vi "peak -- four corner circle transformation logic.vi"(6 "corrected phase":dbl, 7 "4 corner circle transformation":T3=enum."fix phase", 8 "lorentzian in":T1 {"z∞ (V)" format="%#9_9f"; "Q" format="%#9_9f"; "φ (rad)" format="%#9_9f"; "Γ (Hz)" format="%#9_9f"; "f (Hz)" format="%#9_9f"}, 9 "gamma":dbl, 10 "omega":dbl, 11 "circle corners in":T2={"z (-pi/2)"=-1.0311345636926572+0.5736824521422934i, "z(inf)"=-0.5200164984937075+1.0975277942502903i, "z (pi/2)"=-1.0311345636926572+0.5736824521422934i, "z center"=-0.5136528600391839+0.580046090596817i, "z(0)"=-0.5200164984937075+1.0975277942502903i, "radius"=-1.0311345636926572}) -> (0 "lorentzian out":T1={"Amp (VHz)"=-1.0311345636926572, "f (Hz)"=-1.0311345636926572, "Γ (Hz)"=-1.0311345636926572, "φ (rad)"=-1.0311345636926572, "Q"=-1.0311345636926572, "Norm  Ampl"=-1.0311345636926572, "z∞ (V)"=-1.0311345636926572+0.0i, "4corners"={"z (-pi/2)"=-1.0311345636926572+0.5736824521422934i, "z(inf)"=-0.5200164984937075+1.0975277942502903i, "z (pi/2)"=-1.0311345636926572+0.5736824521422934i, "z center"=-0.5136528600391839+0.580046090596817i, "z(0)"=-0.5200164984937075+1.0975277942502903i, "radius"=-1.0311345636926572}} {"z∞ (V)" format="%#9_9f"; "Q" format="%#9_9f"; "φ (rad)" format="%#9_9f"; "Γ (Hz)" format="%#9_9f"; "f (Hz)" format="%#9_9f"}, 3 "circle corners out":T2={"z (-pi/2)"=-1.0311345636926572+0.5736824521422934i, "z(inf)"=-0.5200164984937075+1.0975277942502903i, "z (pi/2)"=-1.0311345636926572+0.5736824521422934i, "z center"=-0.5136528600391839+0.580046090596817i, "z(0)"=-0.5200164984937075+1.0975277942502903i, "radius"=-1.0311345636926572})   [LabVIEW 2017]
uses:
  circle corners.ctl
  four-corner circle transformation.ctl
  lorentzian.ctl
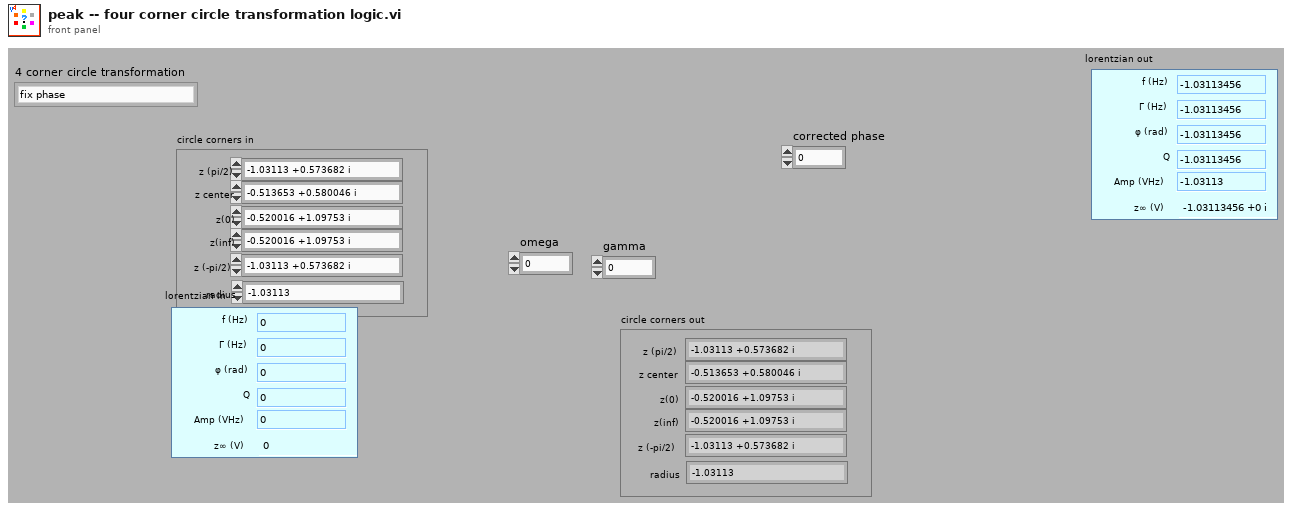
[diagram p1: front panel]
types:
  T1 = typedef "lorentzian.ctl" = cluster{"Amp (VHz)":dbl, "f (Hz)":dbl, "Γ (Hz)":dbl, "φ (rad)":dbl, "Q":dbl, "Norm  Ampl":dbl, "z∞ (V)":cdb, "4corners":T2}
  T2 = typedef "circle corners.ctl" = cluster{"z (-pi/2)":cdb, "z(inf)":cdb, "z (pi/2)":cdb, "z center":cdb, "z(0)":cdb, "radius":dbl}
  T3 = typedef "four-corner circle transformation.ctl" = enum16{"z(c) z(inf)", "z(c) z(zero)", "fix phase", "calculate lorentzian", "z(0) z(+-pi/2)", "shift to zcenter", "to  canonical", "get canonical phase", "get4corners"}
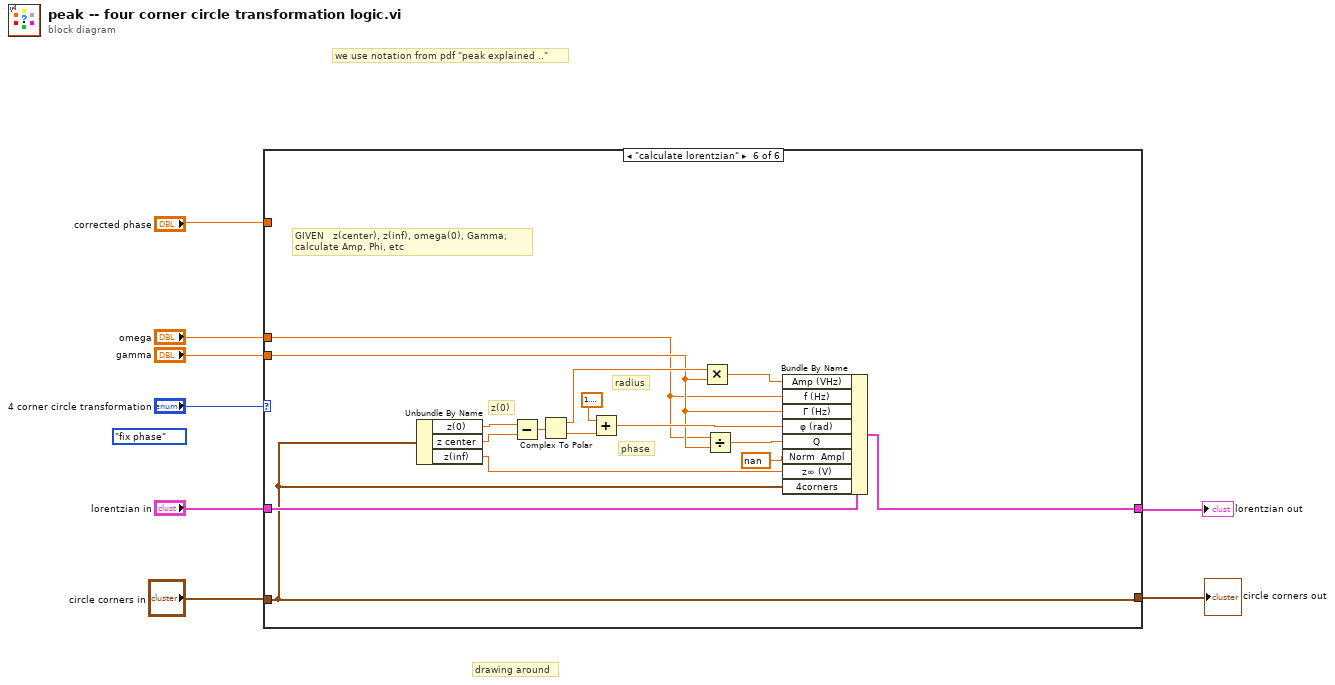
[diagram p0: block diagram]
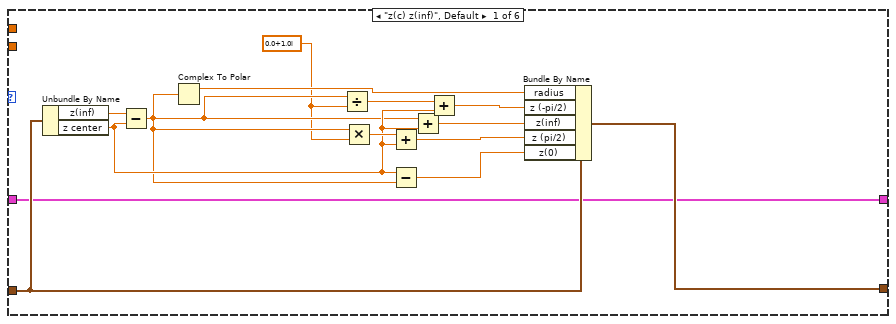
[diagram p2: hidden frame]
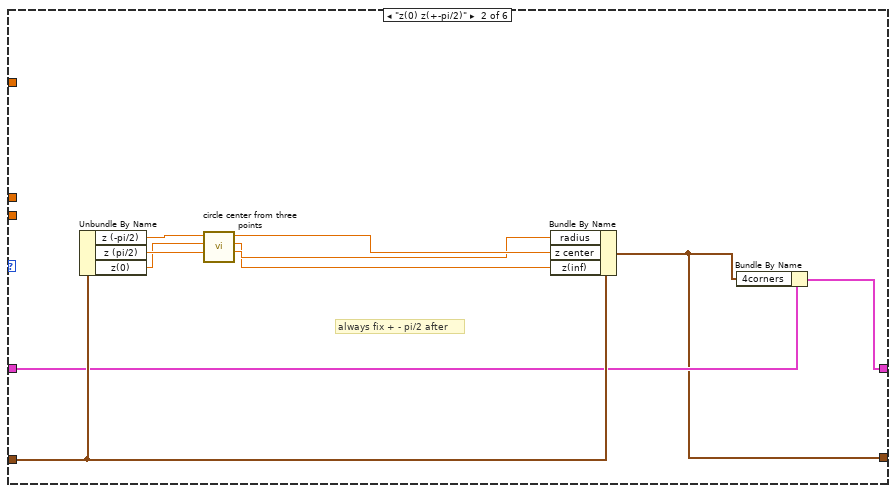
[diagram p3: hidden frame]
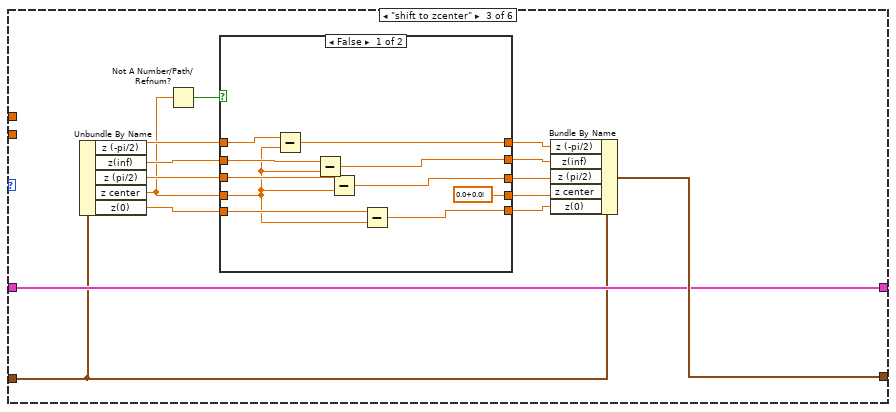
[diagram p4: hidden frame]
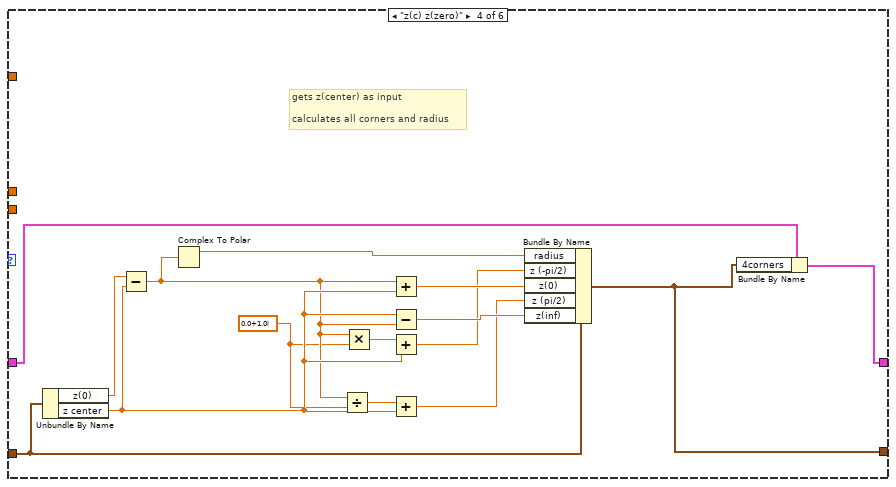
[diagram p6: hidden frame]
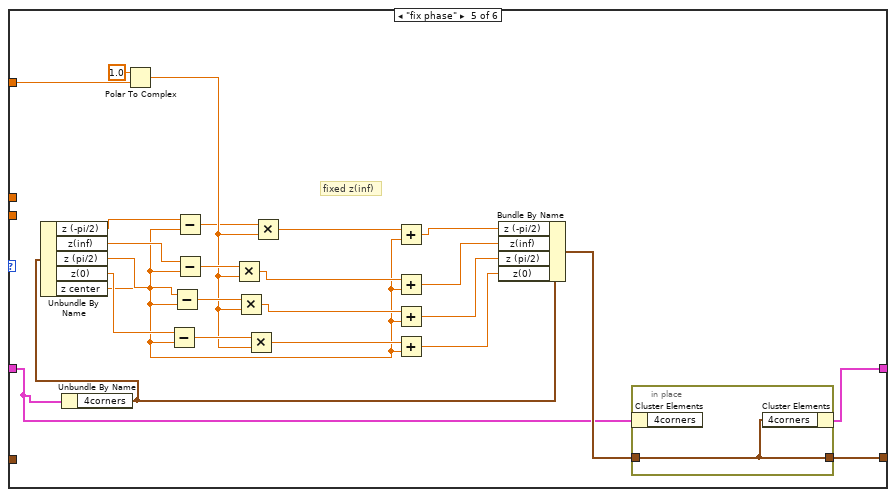
[diagram p7: hidden frame]
diagram:
  (unwired) four-corner_circle_transformation."fix phase" ("4 corner circle transformation")
  # "we use notation from pdf \"peak explained ..\""
  # "drawing around"
  n1 = case shown="\"calculate lorentzian\"" "4 corner circle transformation" {
    tunnel: [w17 w24 w46 w63 w77 w103] -> w8
    tunnel: "circle corners in" -> [w15 w32 w44 w72 _ w103]
    tunnel: "corrected phase" -> [_ _ _ _ w99 _]
    tunnel: "omega" -> [_ _ _ _ _ w106]
    tunnel: "gamma" -> [_ _ _ _ _ w107]
    tunnel: [w9 w23 w45 w62 w80 w104] -> w2
    tunnel: "lorentzian in" -> [w9 w25 w45 w64 w79 w105]
    frame "z(c) z(inf)", Default {
      w10 = cdb 0.0+1.0i ("y")
      n2 = Unbundle By Name(w15) -> ("z(inf)"=w14:cdb, "z center"=w13:cdb)
      n3 = Subtract(x=w14, y=w13) -> (x-y=w12:cdb)
      n4 = Complex To Polar(r * e^(i*theta)=w12) -> (r=w11:dbl)  [unwired: 1 out]
      n5 = Divide(x=w12, y=w10) -> (x/y=w21:cdb)
      n6 = Multiply(x=w12, y=w10) -> (x*y=w22:cdb)
      n7 = Add(x=w22, y=w13) -> (x+y=w18:cdb)
      n8 = Subtract(x=w13, y=w12) -> (x-y=w16:cdb)
      n9 = Add(x=w12, y=w13) -> (x+y=w20:cdb)
      n10 = Add(x=w21, y=w13) -> (x+y=w19:cdb)
      n11 = Bundle By Name(cluster=w15, "radius"=w11, "z (-pi/2)"=w19, "z(inf)"=w20, "z (pi/2)"=w18, "z(0)"=w16) -> (w17:T2)
    }
    frame "z(0) z(+-pi/2)" {
      # "always fix + - pi/2 after"
      n12 = Unbundle By Name(w32) -> ("z (-pi/2)"=w31:cdb, "z (pi/2)"=w30:cdb, "z(0)"=w29:cdb)
      n13 = call "circle center from three points.vi"("z plus"=w30, "z zero"=w29, "z minus"=w31) -> ("radius"=w27:dbl, "z inf"=w26:cdb, "z center"=w28:cdb)  [unwired: 6 in]
      n14 = Bundle By Name(cluster=w32, "radius"=w27, "z center"=w28, "z(inf)"=w26) -> (w24:T2)
      n15 = Bundle By Name(cluster=w25, "4corners"=w24) -> (w23:T1)
    }
    frame "shift to zcenter" {
      n16 = Unbundle By Name(w44) -> ("z (-pi/2)"=w42:cdb, "z(inf)"=w40:cdb, "z (pi/2)"=w38:cdb, "z center"=w34:cdb, "z(0)"=w36:cdb)
      n17 = Not A Number/Path/Refnum?(number/path/refnum=w34) -> (NaN/Path/Refnum?=w33:bool)
      n18 = case shown="False" w33 {
        tunnel: [cdb 0.0+0.0i w58] -> w43
        tunnel: w42 -> [w55 w61]
        tunnel: [w54 w61] -> w41
        tunnel: w40 -> [w53 w60]
        tunnel: [w52 w60] -> w39
        tunnel: w38 -> [w51 w59]
        tunnel: [w50 w59] -> w37
        tunnel: w36 -> [w49 w57]
        tunnel: [w48 w57] -> w35
        tunnel: w34 -> [w47 w58]
        frame False {
          n19 = Subtract(x=w55, y=w47) -> (x-y=w54:cdb)
          n20 = Subtract(x=w53, y=w47) -> (x-y=w52:cdb)
          n21 = Subtract(x=w51, y=w47) -> (x-y=w50:cdb)
          n22 = Subtract(x=w49, y=w47) -> (x-y=w48:cdb)
        }
        frame True {
        }
      }
      n23 = Bundle By Name(cluster=w44, "z (-pi/2)"=w41, "z(inf)"=w39, "z (pi/2)"=w37, "z center"=w43, "z(0)"=w35) -> (w46:T2)
    }
    frame "z(c) z(zero)" {
      w67 = cdb 0.0+1.0i ("y")
      # "gets z(center) as input \n\ncalculates all corners and radius"
      n24 = Unbundle By Name(w72) -> ("z(0)"=w71:cdb, "z center"=w70:cdb)
      n25 = Subtract(x=w71, y=w70) -> (x-y=w69:cdb)
      n26 = Complex To Polar(r * e^(i*theta)=w69) -> (r=w68:dbl)  [unwired: 1 out]
      n27 = Divide(x=w69, y=w67) -> (x/y=w75:cdb)
      n28 = Multiply(x=w69, y=w67) -> (x*y=w76:cdb)
      n29 = Add(x=w69, y=w70) -> (x+y=w74:cdb)
      n30 = Subtract(x=w70, y=w69) -> (x-y=w73:cdb)
      n31 = Add(x=w76, y=w70) -> (x+y=w66:cdb)
      n32 = Add(x=w75, y=w70) -> (x+y=w65:cdb)
      n33 = Bundle By Name(cluster=w72, "radius"=w68, "z (-pi/2)"=w66, "z(0)"=w74, "z (pi/2)"=w65, "z(inf)"=w73) -> (w63:T2)
      n34 = Bundle By Name(cluster=w64, "4corners"=w63) -> (w62:T1)
    }
    frame "fix phase" {
      # "fixed z(inf)"
      n35 = Unbundle By Name(w79) -> ("4corners"=w78:T2)
      n36 = Unbundle By Name(w78) -> ("z (-pi/2)"=w101:cdb, "z(inf)"=w98:cdb, "z (pi/2)"=w97:cdb, "z(0)"=w96:cdb, "z center"=w86:cdb)
      n37 = Polar To Complex(1:w99, 2:1.0 ("r")) -> (0:w92:cdb)
      n38 = Subtract(x=w96, y=w86) -> (x-y=w95:cdb)
      n39 = Subtract(x=w97, y=w86) -> (x-y=w94:cdb)
      n40 = Subtract(x=w101, y=w86) -> (x-y=w91:cdb)
      n41 = Subtract(x=w98, y=w86) -> (x-y=w93:cdb)
      n42 = Multiply(x=w93, y=w92) -> (x*y=w89:cdb)
      n43 = Multiply(x=w94, y=w92) -> (x*y=w88:cdb)
      n44 = Multiply(x=w95, y=w92) -> (x*y=w87:cdb)
      n45 = Multiply(x=w91, y=w92) -> (x*y=w90:cdb)
      n46 = Add(x=w90, y=w86) -> (x+y=w85:cdb)
      n47 = Add(x=w89, y=w86) -> (x+y=w84:cdb)
      n48 = Add(x=w88, y=w86) -> (x+y=w83:cdb)
      n49 = Add(x=w87, y=w86) -> (x+y=w82:cdb)
      n50 = Bundle By Name(cluster=w78, "z (-pi/2)"=w85, "z(inf)"=w84, "z (pi/2)"=w83, "z(0)"=w82) -> (w81:T2)
      n51 = in-place {
        in-place-border: w81 -> [w102]
        in-place-border: [w102] -> w77
        n52 = in-place-cluster #1(w79) -> ()  [unwired: 1 out]
        n53 = in-place-cluster #1("4corners"=w102) -> (w80:T1)
      }
    }
    frame "calculate lorentzian" {
      # "z(0)"
      # "radius"
      # "phase"
      # "GIVEN   z(center), z(inf), omega(0), Gamma, \ncalculate Amp, Phi, etc"
      n54 = Unbundle By Name(w103) -> ("z(0)"=w108:cdb, "z center"=w118:cdb, "z(inf)"=w117:cdb)
      n55 = Subtract(x=w108, y=w118) -> (x-y=w116:cdb)
      n56 = Complex To Polar(r * e^(i*theta)=w116) -> (r=w111:dbl, theta=w114:dbl)
      n57 = Add(x=1.5707963267948966, y=w114) -> (x+y=w113:dbl)
      n58 = Multiply(x=w111, y=w107) -> (x*y=w110:dbl)
      n59 = Divide(x=w106, y=w107) -> (x/y=w112:dbl)
      n60 = Bundle By Name(cluster=w105, "Amp (VHz)"=w110, "f (Hz)"=w106, "Γ (Hz)"=w107, "φ (rad)"=w113, "Q"=w112, "Norm  Ampl"=nan, "z∞ (V)"=w117, "4corners"=w103) -> (w104:T1)
    }
  }
  "circle corners out" <- w8
  "lorentzian out" <- w2
